vi "FTW-Package-Lossy-CreateQueue.vi"(9 "max queue size (1)":i32=1, 11 "error in":errorcluster) -> (4 "Queue":refnum<queue>, 15 "error out":errorcluster)   [LabVIEW 2013, in "FTW-Package-Lossy.lvclass"]
uses:
  FTW-Package-Lossy.lvclass
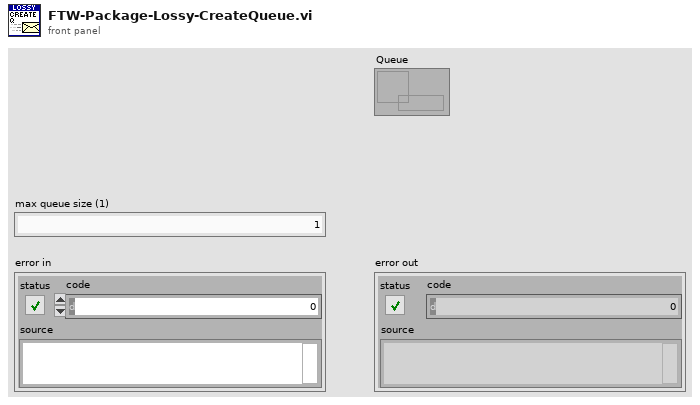
[diagram p1: front panel]
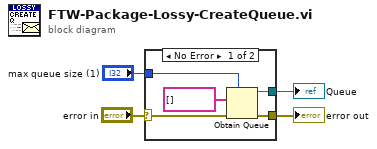
[diagram p0: block diagram]
diagram:
  n1 = case shown="No Error" "error in" {
    selector: "error in" -> [w9 w10]
    tunnel: [w8 w10] -> w3
    tunnel: [w7 _] -> w2
    tunnel: "max queue size (1)" -> [w5 _]
    frame No Error {
      n2 = Obtain Queue(max queue size (-1, unlimited)=w5, element data type=string[] [] ("Parts"), error in (no error)=w9) -> (queue out=w7:refnum<queue>, error out=w8:errorcluster)  [unwired: 2 in, 1 out]
    }
    frame Error {
    }
  }
  "error out" <- w3
  "Queue" <- w2
